vi "实时小时数据单参数上传.vi"(11 "错误输入（无错误）":errorcluster) -> (4 "数据发送起始时间":timestamp format="%<%.3X\n%Y/%m/%d>T", 15 "error out":errorcluster)   [LabVIEW 2016, in "数据传输系统-06.lvlib"]
uses:
  <vilib>/Utility/config.llb/Read Key (String).vi
  <vilib>/Utility/config.llb/Write Key (String).vi
  <vilib>/Utility/config.llb/NI_LVConfig.lvlib
panel:
  out "数据拆分":bool
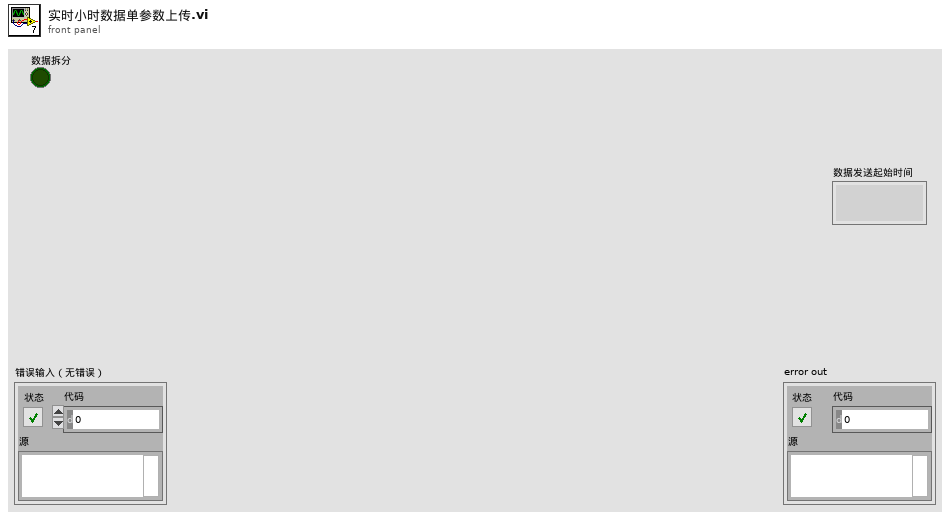
[diagram p1: front panel]
types:
  T1 = cluster{"CODMn":string, "CODCr":string, "DO":string, "铜":string, "PH":string, "氨氮":string, "比电导率":string, "水温":string, "COD":string, "浊度":string, "总氮":string, "总磷":string, "叶绿素a":string, "藻密度":string, "水位":string, "流速":string, "瞬时流量":string, "累积流量":string, "亚硝酸盐":string, "硫化物":string, "ORP":string, "铅":string, "镉":string, "锌":string, "镍":string, "锰":string, "汞":string, "气温":string, "气压":string, "风速":string, "风向":string, "盐度":string, "磷酸盐":string, "硝氮":string, "氟化物":string, "挥发酚":string, "氯化物":string}
  T2 = cluster{"setini":string, "sysini":string, "hechaini":string, "actualwrite":string, "actualread":string, "datasent":string, "反控命令信息队列":string, "反控与仪器交互":string}
  T3 = typedef "NI_LVConfig.lvlib/Config Data RefNum.ctl" = refnum<k1>
  T4 = cluster{"time1":string, "time2":string, "time3":string, "time4":string, "time5":string, "time6":string, "time7":string, "time8":string, "time9":string, "time10":string, "time11":string, "time12":string, "time13":string, "time14":string, "time15":string, "time16":string, "time17":string, "time18":string, "time19":string, "time20":string, "time21":string, "time22":string, "time23":string, "time24":string, "time25":string, "time26":string, "time27":string, "time28":string, "time29":string, "time30":string, "time31":string, "time32":string, "time33":string, "time34":string, "time35":string, "time36":string, "time37":string}
  T5 = cluster{"水样数据索引[0]":string, "水样数据索引[1]":string, "水样数据索引[2]":string, "水样数据索引[3]":string, "水样数据索引[4]":string, "水样数据索引[5]":string, "水样数据索引[6]":string, "水样数据索引[7]":string, "水样数据索引[8]":string, "水样数据索引[9]":string, "水样数据索引[10]":string, "水样数据索引[11]":string, "水样数据索引[12]":string, "水样数据索引[13]":string, "水样数据索引[14]":string, "水样数据索引[15]":string, "水样数据索引[16]":string, "水样数据索引[17]":string, "水样数据索引[18]":string, "水样数据索引[19]":string, "水样数据索引[20]":string, "水样数据索引[21]":string, "水样数据索引[22]":string, "水样数据索引[23]":string, "水样数据索引[24]":string, "水样数据索引[25]":string, "水样数据索引[26]":string, "水样数据索引[27]":string, "水样数据索引[28]":string, "水样数据索引[29]":string, "水样数据索引[30]":string, "水样数据索引[31]":string, "水样数据索引[32]":string, "水样数据索引[33]":string, "水样数据索引[34]":string, "水样数据索引[35]":string, "水样数据索引[36]":string}
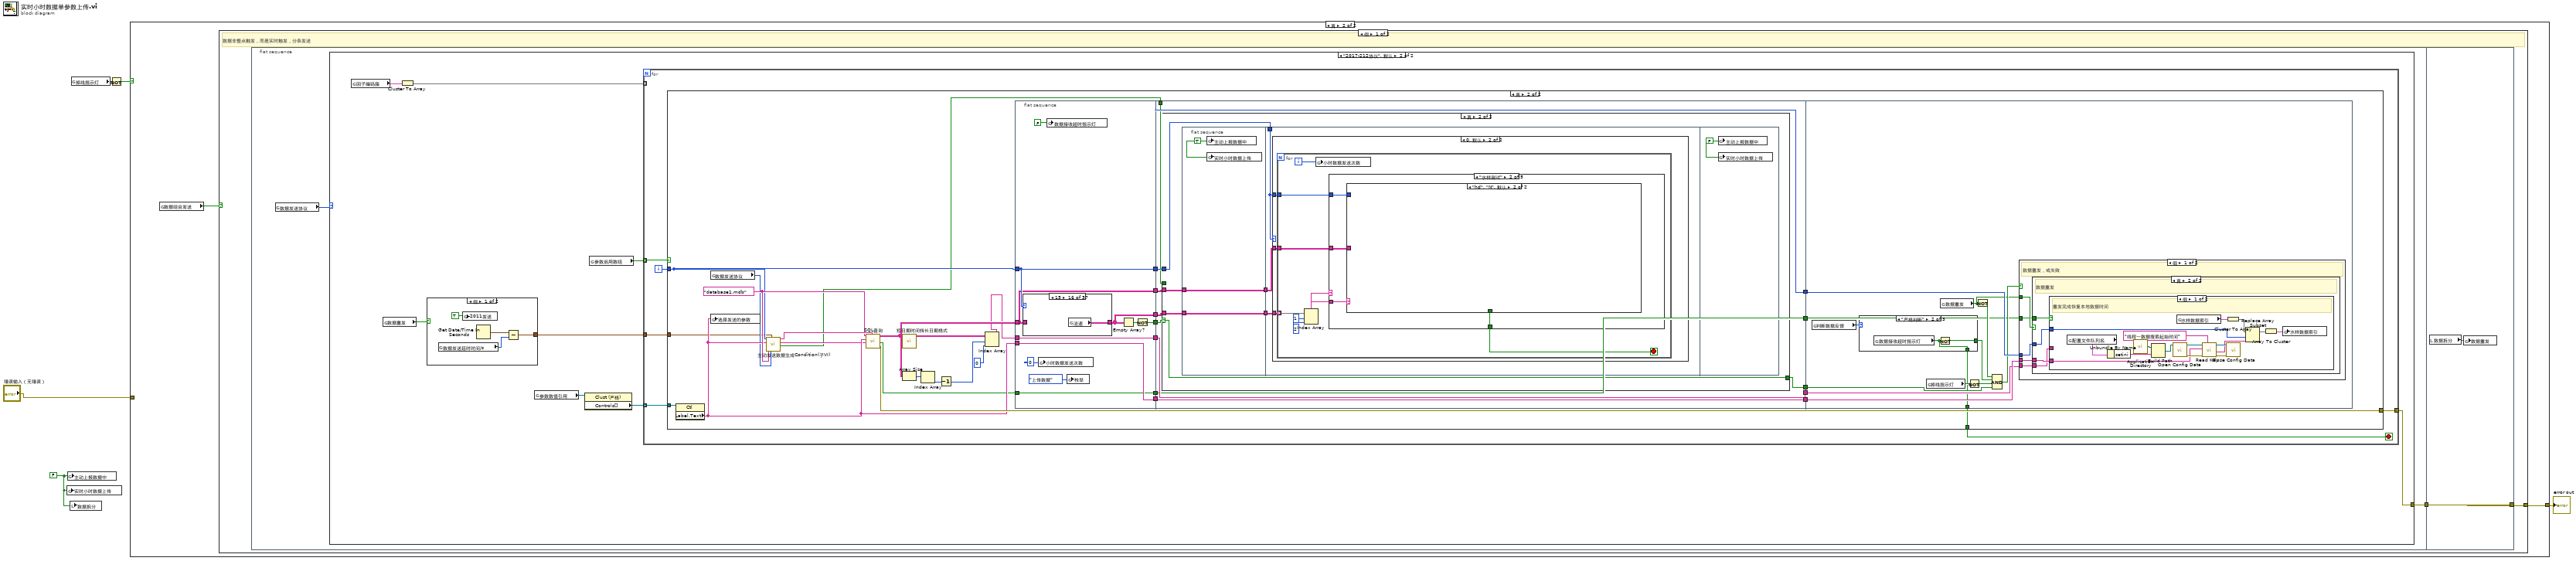
[diagram p0: block diagram]
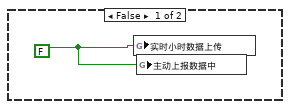
[diagram p2: hidden frame]
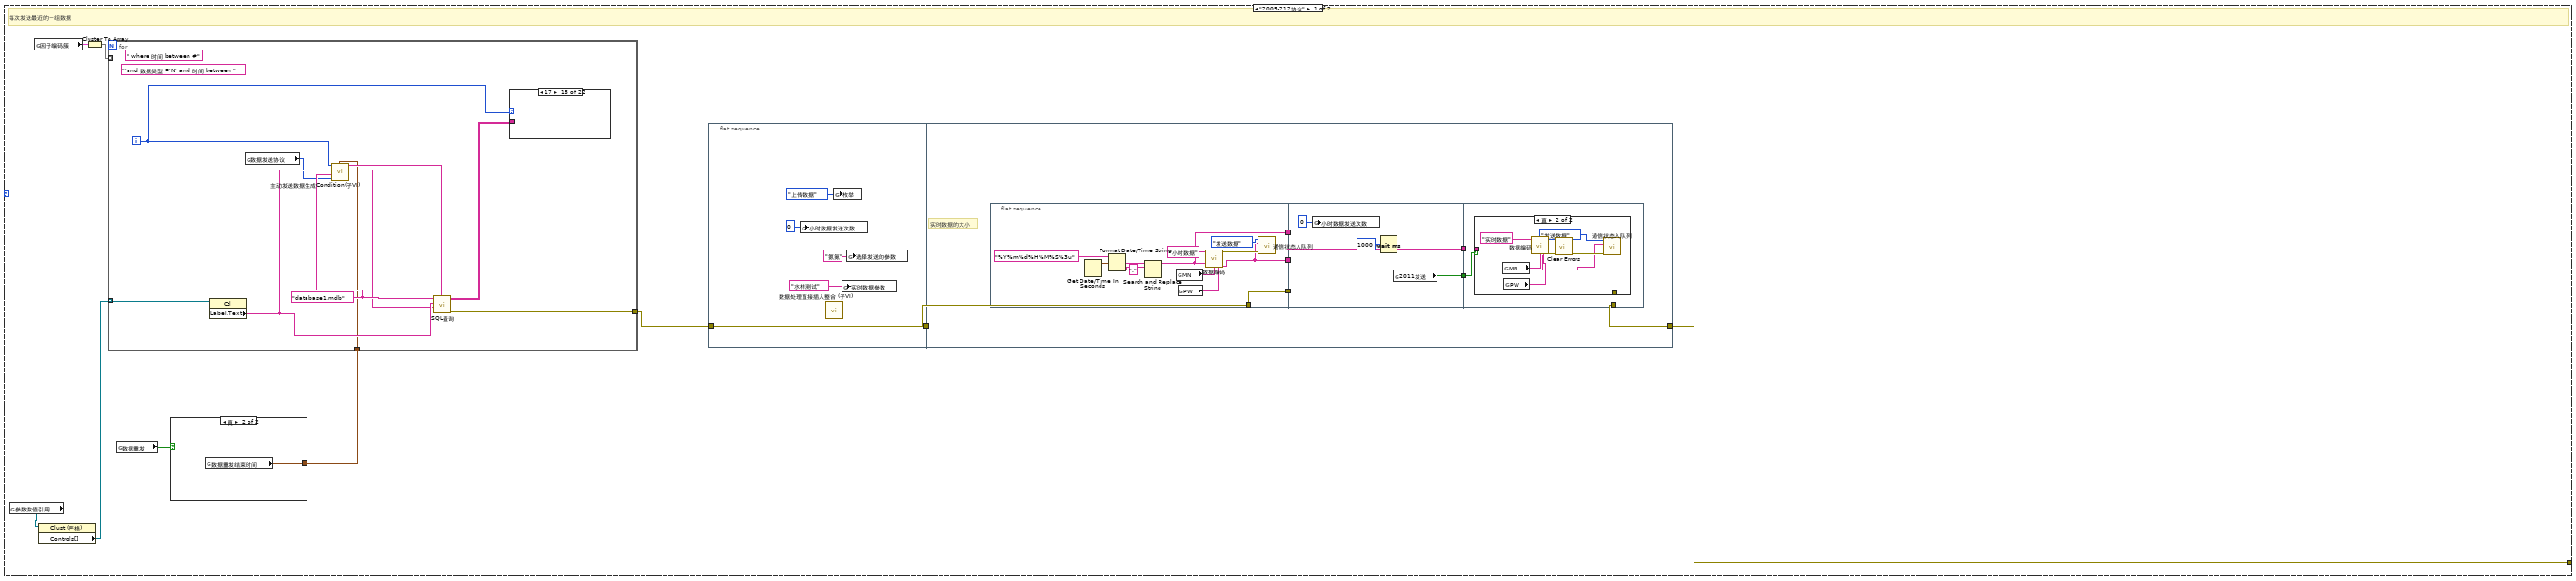
[diagram p3: hidden frame]
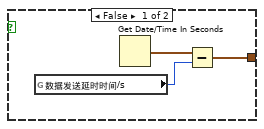
[diagram p4: hidden frame]
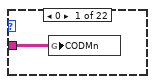
[diagram p6: hidden frame]
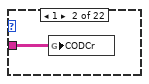
[diagram p7: hidden frame]
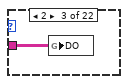
[diagram p8: hidden frame]
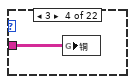
[diagram p9: hidden frame]
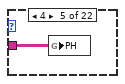
[diagram p10: hidden frame]
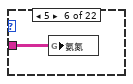
[diagram p11: hidden frame]
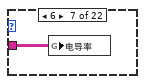
[diagram p12: hidden frame]
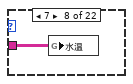
[diagram p13: hidden frame]
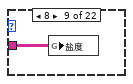
[diagram p14: hidden frame]
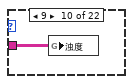
[diagram p15: hidden frame]
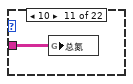
[diagram p16: hidden frame]
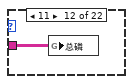
[diagram p17: hidden frame]
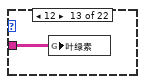
[diagram p18: hidden frame]
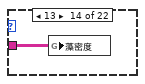
[diagram p19: hidden frame]
diagram:
  w1 = FALSE ("小时数据上传")
  n1 = global write "全局1.vi" "实时小时数据上传"(w1) -> ()
  n2 = global write "全局 数据发送重叠.vi" "主动上报数据中"(w1) -> ()
  n3 = local write "数据拆分"(w1) -> ()
  n4 = global read "全局 数据发送重叠.vi" "掉线指示灯"() -> (w5:bool)
  n5 = Not(x=w5) -> (.not. x?=w4:bool)
  n6 = case shown="真" w4 {
    tunnel: [_ w8] -> w3
    tunnel: "错误输入（无错误）" -> [_ _]
    frame False {
      w6 = FALSE ("小时数据上传")
      n7 = global write "全局1.vi" "实时小时数据上传"(w6) -> ()
      n8 = global write "全局 数据发送重叠.vi" "主动上报数据中"(w6) -> ()
    }
    frame True {
      n9 = global read "断电保存全局.vi" "数据组合发送"() -> (w7:bool)
      n10 = case shown="假" w7 {
        tunnel: [w9 _] -> w8
        frame False {
          # "数据非整点触发，而是实时触发，分条发送"
          n11 = flat-sequence {
            tunnel: [w12] -> w10
            tunnel: [w370] -> w9
            tunnel: w10 -> [w370]
            frame #0 {
              n12 = global read "断电保存全局.vi" "数据发送协议"() -> (w11:enum16{"2005-212协议", "2017-212协议"})
              n13 = case shown="\"2017-212协议\", 默认" w11 {
                tunnel: [w17 w99] -> w12
                frame "2005-212协议" {
                  # "每次发送最近的一组数据"
                  n14 = global read "断电保存全局.vi" "参数数值引用"() -> (w15:refnum<vi>)
                  n15 = global read "断电保存全局.vi" "因子编码簇"() -> (w16:T1)
                  n16 = property class="Clust (严格)"(reference=w15) -> ("Controls[]"=w18:refnum<vi>[])  [unwired: 1 in, 2 out]
                  n17 = Cluster To Array(cluster=w16) -> (array=w21:string[])
                  n18 = global read "断电保存全局.vi" "数据重发"() -> (w14:bool)
                  n19 = case shown="真" w14 {
                    tunnel: [w22 w25] -> w13
                    frame False {
                      n20 = global read "断电保存全局.vi" "数据发送延时时间/s"() -> (w23:i32)
                      n21 = Get Date/Time In Seconds() -> (seconds since 1Jan1904=w24:timestamp)
                      n22 = Subtract(x=w24, y=w23) -> (x-y=w22:timestamp)
                    }
                    frame True {
                      n23 = global read "断电保存全局.vi" "数据重发结束时间"() -> (w25:timestamp)
                    }
                  }
                  n24 = for {
                    tunnel: w21 -> [_] mode=indexing
                    tunnel: [w75] -> w20
                    tunnel: w18 -> [w70] mode=indexing
                    tunnel: w13 -> [w67]
                    i -> [w68]
                    (unwired) " where 时间 between #"
                    w73 = "database1.mdb" ("database")
                    (unwired) "'and 数据类型 ='N' and 时间 between "
                    n25 = property class="Ctl"(reference=w70) -> ("Label.Text"=w74:string)  [unwired: 1 in, 2 out]
                    n26 = global read "断电保存全局.vi" "数据发送协议"() -> (w71:enum16{"2005-212协议", "2017-212协议"})
                    n27 = call "主动发送数据生成Condition(子VI).vi"("结束时间"=w67, "数据发送协议"=w71, "database"=w73, "Label.Text"=w74, "数值"=w68) -> ("columns"=w66:string[], "CONDITION"=w72:string)  [unwired: 3 in, 2 out]
                    n28 = call "SQL查询.vi"("condition"=w72, "columns"=w66, "table输入"=w74, "database"=w73) -> ("error out"=w75:errorcluster, "data"=w69:string[][])  [unwired: 4 in, 2 out]
                    n29 = case shown="17" w68 {
                      tunnel: w69 -> [w76 w77 w78 w79 w80 w81 w82 w83 w84 w85 w86 w87 w88 w89 _ _ _ _ w90 w91 w92 _]
                      frame 0 {
                        n30 = global write "全局 所有参数.vi" "CODMn"(w76) -> ()
                      }
                      frame 1 {
                        n31 = global write "全局 所有参数.vi" "CODCr"(w77) -> ()
                      }
                      frame 2 {
                        n32 = global write "全局 所有参数.vi" "DO"(w78) -> ()
                      }
                      frame 3 {
                        n33 = global write "全局 所有参数.vi" "铜"(w79) -> ()
                      }
                      frame 4 {
                        n34 = global write "全局 所有参数.vi" "PH"(w80) -> ()
                      }
                      frame 5 {
                        n35 = global write "全局 所有参数.vi" "氨氮"(w81) -> ()
                      }
                      frame 6 {
                        n36 = global write "全局 所有参数.vi" "电导率"(w82) -> ()
                      }
                      frame 7 {
                        n37 = global write "全局 所有参数.vi" "水温"(w83) -> ()
                      }
                      frame 8 {
                        n38 = global write "全局 所有参数.vi" "盐度"(w84) -> ()
                      }
                      frame 9 {
                        n39 = global write "全局 所有参数.vi" "浊度"(w85) -> ()
                      }
                      frame 10 {
                        n40 = global write "全局 所有参数.vi" "总氮"(w86) -> ()
                      }
                      frame 11 {
                        n41 = global write "全局 所有参数.vi" "总磷"(w87) -> ()
                      }
                      frame 12 {
                        n42 = global write "全局 所有参数.vi" "叶绿素"(w88) -> ()
                      }
                      frame 13 {
                        n43 = global write "全局 所有参数.vi" "藻密度"(w89) -> ()
                      }
                      frame 14 {
                      }
                      frame 15 {
                      }
                      frame 16 {
                      }
                      frame 17 {
                      }
                      frame 18 {
                        n44 = global write "全局 所有参数.vi" "亚硝酸盐"(w90) -> ()
                      }
                      frame 19 {
                        n45 = global write "全局 所有参数.vi" "硫化物"(w91) -> ()
                      }
                      frame 20 {
                        n46 = global write "全局 所有参数.vi" "ORP"(w92) -> ()
                      }
                      frame 21, Default {
                      }
                    }
                  }
                  n47 = flat-sequence {
                    tunnel: w20 -> [w26]
                    tunnel: [w26] -> w19
                    tunnel: w19 -> [w35]
                    tunnel: [w34] -> w17
                    frame #0 {
                      n48 = global write "全局 小时数据发送次数.vi" "小时数据发送次数"(0 ("小时数据发送次数")) -> ()
                      n49 = call "数据处理直接插入整合 (子VI).vi"() -> ()  [unwired: 12 in]
                      n50 = global write "全局1.vi" "枚举"(enum16{"返回请求应答", "上传数据", "返回执行结果"}."上传数据" ("枚举")) -> ()
                      n51 = global write "全局 实时数据参数.vi" "实时数据参数"("水样测试" ("实时数据参数")) -> ()
                      n52 = global write "全局 水样时间.vi" "选择发送的参数"("氨氮" ("选择发送的参数")) -> ()
                    }
                    frame #1 {
                      # "实时数据的大小"
                      n53 = flat-sequence {
                        tunnel: [w38] -> w37
                        tunnel: [w41] -> w36
                        tunnel: w35 -> [w41]
                        tunnel: [w40] -> w33
                        tunnel: w37 -> [_]
                        tunnel: w36 -> [_]
                        tunnel: w33 -> [w51]
                        tunnel: [w51] -> w32
                        tunnel: [w50] -> w31
                        tunnel: [w56] -> w34
                        tunnel: w32 -> [w55]
                        tunnel: w31 -> [w54]
                        frame #0 {
                          n54 = Get Date/Time In Seconds() -> (seconds since 1Jan1904=w47:timestamp)
                          n55 = Format Date/Time String(time format string (%c)="%Y%m%d%H%M%S%3u" ("时间格式字符串(%c)"), seconds (now)=w47) -> (date/time string=w48:string)  [unwired: 1 in]
                          n56 = Search and Replace String(input string=w48, search string="." ("搜索字符串")) -> (result string=w40:string)  [unwired: 6 in, 3 out]
                          n57 = global read "断电保存全局.vi" "MN"() -> (w44:string)
                          n58 = global read "断电保存全局.vi" "PW"() -> (w43:string)
                          n59 = call "数据编码.vi"("table输入"="小时数据" ("新元素/子数组"), "QN"=w40, "MN"=w44, "PW"=w43) -> ("错误常量"=w42:errorcluster, "通讯包字符串"=w38:string)  [unwired: 10 in]
                          n60 = call "通信状态入队列.vi"("错误输入（无错误）"=w42, "发送报文"=w38, "枚举"=enum16{"打开连接", "发送数据", "读取数据", "数据处理", "关闭连接"}."发送数据") -> ()  [unwired: 8 in, 1 out]
                        }
                        frame #1 {
                          n61 = global write "全局 小时数据发送次数.vi" "小时数据发送次数"(0 ("小时数据发送次数")) -> ()
                          n62 = Wait (ms)(milliseconds to wait=u32 1000 ("等待时间（毫秒）")) -> ()  [unwired: 1 out]
                          n63 = global read "断电保存全局.vi" "2011发送"() -> (w50:bool)
                        }
                        frame #2 {
                          n64 = case shown="真" w54 {
                            tunnel: [_ w61] -> w56
                            tunnel: w55 -> [_ w60]
                            frame False {
                            }
                            frame True {
                              n65 = global read "断电保存全局.vi" "MN"() -> (w63:string)
                              n66 = global read "断电保存全局.vi" "PW"() -> (w64:string)
                              n67 = call "数据编码.vi"("table输入"="实时数据" ("新元素/子数组"), "QN"=w60, "MN"=w63, "PW"=w64) -> ("错误常量"=w62:errorcluster, "通讯包字符串"=w57:string)  [unwired: 10 in]
                              n68 = call <vilib>:"Clear Errors.vi"("error in (no error)"=w62) -> ("error out"=w59:errorcluster)  [unwired: 5 in, 1 out]
                              n69 = call "通信状态入队列.vi"("错误输入（无错误）"=w59, "发送报文"=w57, "枚举"=enum16{"打开连接", "发送数据", "读取数据", "数据处理", "关闭连接"}."发送数据") -> ("错误输出"=w61:errorcluster)  [unwired: 8 in]
                            }
                          }
                        }
                      }
                    }
                  }
                }
                frame "2017-212协议", Default {
                  n70 = global read "断电保存全局.vi" "因子编码簇"() -> (w97:T1)
                  n71 = global read "断电保存全局.vi" "数据重发"() -> (w94:bool)
                  n72 = Cluster To Array(cluster=w97) -> (array=w100:string[])
                  n73 = case shown="假" w94 {
                    tunnel: [w102 w105] -> w93
                    frame False {
                      n74 = global read "断电保存全局.vi" "数据发送延时时间/s"() -> (w103:i32)
                      n75 = global write "断电保存全局.vi" "2011发送"(TRUE ("2011发送")) -> ()
                      n76 = Get Date/Time In Seconds() -> (seconds since 1Jan1904=w104:timestamp)
                      n77 = Subtract(x=w104, y=w103) -> (x-y=w102:timestamp)
                    }
                    frame True {
                      n78 = global read "断电保存全局.vi" "数据重发结束时间"() -> (w105:timestamp)
                    }
                  }
                  n79 = global read "断电保存全局.vi" "参数数值引用"() -> (w96:refnum<vi>)
                  n80 = property class="Clust (严格)"(reference=w96) -> ("Controls[]"=w98:refnum<vi>[])  [unwired: 1 in, 2 out]
                  n81 = global read "断电保存全局.vi" "参数启用数组"() -> (w95:bool[])
                  n82 = for {
                    tunnel: w100 -> [_] mode=indexing
                    tunnel: [w111] -> w99
                    tunnel: w98 -> [w109] mode=indexing
                    tunnel: w95 -> [w108] mode=indexing
                    tunnel: w93 -> [w107]
                    i -> [w110]
                    stop <- w106 stop-if-true
                    n83 = case shown="真" w108 {
                      tunnel: [_ w132] -> w111
                      tunnel: w110 -> [_ w123]
                      tunnel: w109 -> [_ w122]
                      tunnel: w107 -> [_ w119]
                      tunnel: [_ w117] -> w106
                      frame False {
                      }
                      frame True {
                        w131 = "database1.mdb" ("database")
                        n84 = property class="Ctl"(reference=w122) -> ("Label.Text"=w130:string)  [unwired: 1 in, 2 out]
                        n85 = global read "断电保存全局.vi" "数据发送协议"() -> (w129:enum16{"2005-212协议", "2017-212协议"})
                        n86 = global write "全局 水样时间.vi" "选择发送的参数"(w130) -> ()
                        n87 = call "主动发送数据生成Condition(子VI).vi"("结束时间"=w119, "数据发送协议"=w129, "database"=w131, "Label.Text"=w130, "数值"=w123) -> ("database溢出"=w112:bool, "columns"=w121:string[], "CONDITION"=w134:string)  [unwired: 3 in, 1 out]
                        n88 = call "SQL查询.vi"("condition"=w134, "columns"=w121, "table输入"=w130, "database"=w131) -> ("error out"=w132:errorcluster, "拆分数据"=w115:bool, "data"=w126:string[][])  [unwired: 4 in, 1 out]
                        n89 = call "短日期时间转长日期格式.vi"("data"=w126) -> ("输出数组"=w133:string[][])  [unwired: 10 in]
                        n90 = Array Size(array=w126) -> (size(s)=w128:i32[])
                        n91 = Index Array(array=w128) -> (element=w127:i32)  [unwired: 1 in]
                        n92 = Decrement(x=w127) -> (x-1=w125:i32)
                        n93 = Index Array(array=w133, index (row)=w125, index (col)=0 ("禁用的索引 (列)")) -> (element=w113:string)
                        n94 = flat-sequence {
                          tunnel: [w146] -> w142
                          tunnel: [w145] -> w141
                          tunnel: w126 -> [w144]
                          tunnel: w123 -> [w149]
                          tunnel: w130 -> [w151]
                          tunnel: [w151] -> w140
                          tunnel: w113 -> [w150]
                          tunnel: [w150] -> w139
                          tunnel: [w149] -> w138
                          tunnel: [w144] -> w118
                          tunnel: [w143] -> w116
                          tunnel: w115 -> [w143]
                          tunnel: w142 -> [w195]
                          tunnel: w141 -> [w199]
                          tunnel: [w198] -> w137
                          tunnel: w140 -> [w198]
                          tunnel: [w197] -> w136
                          tunnel: w139 -> [w197]
                          tunnel: [w196] -> w135
                          tunnel: w138 -> [w196]
                          tunnel: [w192] -> w120
                          tunnel: w118 -> [w194]
                          tunnel: w116 -> [w193]
                          tunnel: [w193] -> w114
                          tunnel: w112 -> [w191]
                          tunnel: w137 -> [w310]
                          tunnel: w136 -> [w309]
                          tunnel: w135 -> [w308]
                          tunnel: w120 -> [w307]
                          tunnel: [w299] -> w117
                          tunnel: w114 -> [w298]
                          frame #0 {
                            n95 = case shown="15" w149 {
                              tunnel: w144 -> [w154 w155 w156 w157 w158 w159 w160 w161 w162 w163 w164 w165 w166 w167 _ _ _ _ w172 w173 w174 w175 w176 w177 w178 w179 w180 _ _ _ _ w185 w186 w187 w188 w189 w190]
                              tunnel: [w154 w155 w156 w157 w158 w159 w160 w161 w162 w163 w164 w165 w166 w167 w168 w169 w170 w171 w172 w173 w174 w175 w176 w177 w178 w179 w180 w181 w182 w183 w184 w185 w186 w187 w188 w189 w190] -> w145
                              frame 0, Default {
                                n96 = global write "全局 所有参数.vi" "CODMn"(w154) -> ()
                              }
                              frame 1 {
                                n97 = global write "全局 所有参数.vi" "CODCr"(w155) -> ()
                              }
                              frame 2 {
                                n98 = global write "全局 所有参数.vi" "DO"(w156) -> ()
                              }
                              frame 3 {
                                n99 = global write "全局 所有参数.vi" "铜"(w157) -> ()
                              }
                              frame 4 {
                                n100 = global write "全局 所有参数.vi" "PH"(w158) -> ()
                              }
                              frame 5 {
                                n101 = global write "全局 所有参数.vi" "氨氮"(w159) -> ()
                              }
                              frame 6 {
                                n102 = global write "全局 所有参数.vi" "电导率"(w160) -> ()
                              }
                              frame 7 {
                                n103 = global write "全局 所有参数.vi" "水温"(w161) -> ()
                              }
                              frame 8 {
                                n104 = global write "全局 所有参数.vi" "盐度"(w162) -> ()
                              }
                              frame 9 {
                                n105 = global write "全局 所有参数.vi" "浊度"(w163) -> ()
                              }
                              frame 10 {
                                n106 = global write "全局 所有参数.vi" "总氮"(w164) -> ()
                              }
                              frame 11 {
                                n107 = global write "全局 所有参数.vi" "总磷"(w165) -> ()
                              }
                              frame 12 {
                                n108 = global write "全局 所有参数.vi" "叶绿素"(w166) -> ()
                              }
                              frame 13 {
                                n109 = global write "全局 所有参数.vi" "藻密度"(w167) -> ()
                              }
                              frame 14 {
                                n110 = global read "全局 所有参数.vi" "水位"() -> (w168:string[][])
                              }
                              frame 15 {
                                n111 = global read "全局 所有参数.vi" "流速"() -> (w169:string[][])
                              }
                              frame 16 {
                                n112 = global read "全局 所有参数.vi" "瞬时流量"() -> (w170:string[][])
                              }
                              frame 17 {
                                n113 = global read "全局 所有参数.vi" "累积流量"() -> (w171:string[][])
                              }
                              frame 18 {
                                n114 = global write "全局 所有参数.vi" "亚硝酸盐"(w172) -> ()
                              }
                              frame 19 {
                                n115 = global write "全局 所有参数.vi" "硫化物"(w173) -> ()
                              }
                              frame 20 {
                                n116 = global write "全局 所有参数.vi" "ORP"(w174) -> ()
                              }
                              frame 21 {
                                n117 = global write "全局 所有参数.vi" "铅"(w175) -> ()
                              }
                              frame 22 {
                                n118 = global write "全局 所有参数.vi" "镉"(w176) -> ()
                              }
                              frame 23 {
                                n119 = global write "全局 所有参数.vi" "锌"(w177) -> ()
                              }
                              frame 24 {
                                n120 = global write "全局 所有参数.vi" "镍"(w178) -> ()
                              }
                              frame 25 {
                                n121 = global write "全局 所有参数.vi" "锰"(w179) -> ()
                              }
                              frame 26 {
                                n122 = global write "全局 所有参数.vi" "汞"(w180) -> ()
                              }
                              frame 27 {
                                n123 = global read "全局 所有参数.vi" "气温"() -> (w181:string[][])
                              }
                              frame 28 {
                                n124 = global read "全局 所有参数.vi" "气压"() -> (w182:string[][])
                              }
                              frame 29 {
                                n125 = global read "全局 所有参数.vi" "风速"() -> (w183:string[][])
                              }
                              frame 30 {
                                n126 = global read "全局 所有参数.vi" "风向"() -> (w184:string[][])
                              }
                              frame 31 {
                                n127 = global write "全局 所有参数.vi" "盐度 2"(w185) -> ()
                              }
                              frame 32 {
                                n128 = global write "全局 所有参数.vi" "磷酸盐"(w186) -> ()
                              }
                              frame 33 {
                                n129 = global write "全局 所有参数.vi" "硝氮"(w187) -> ()
                              }
                              frame 34 {
                                n130 = global write "全局 所有参数.vi" "氟化物"(w188) -> ()
                              }
                              frame 35 {
                                n131 = global write "全局 所有参数.vi" "挥发酚"(w189) -> ()
                              }
                              frame 36 {
                                n132 = global write "全局 所有参数.vi" "氯化物"(w190) -> ()
                              }
                            }
                            n133 = global write "全局 小时数据发送次数.vi" "小时数据发送次数"(0 ("小时数据发送次数")) -> ()
                            n134 = global write "全局 数据发送重叠.vi" "数据接收超时指示灯"(FALSE ("数据接收超时指示灯")) -> ()
                            n135 = global write "全局1.vi" "枚举"(enum16{"返回请求应答", "上传数据", "返回执行结果"}."上传数据" ("枚举")) -> ()
                            n136 = Empty Array?(array=w145) -> (empty?=w147:bool)
                            n137 = Not(x=w147) -> (.not. x?=w146:bool)
                          }
                          frame #1 {
                            n138 = case shown="真" w195 {
                              selector: w195 -> [_ w201]
                              tunnel: w199 -> [_ w206]
                              tunnel: w196 -> [_ w205]
                              tunnel: w194 -> [_ w203]
                              tunnel: [w200 w201] -> w192
                              tunnel: w191 -> [w200 _]
                              frame False {
                              }
                              frame True {
                                n139 = flat-sequence {
                                tunnel: w206 -> [w209]
                                tunnel: [w209] -> w204
                                tunnel: w203 -> [w207]
                                tunnel: [w207] -> w202
                                tunnel: w205 -> [w211]
                                tunnel: w204 -> [w212]
                                tunnel: w202 -> [w210]
                                frame #0 {
                                w208 = TRUE ("小时数据上传")
                                n140 = global write "全局 数据发送重叠.vi" "主动上报数据中"(w208) -> ()
                                n141 = global write "全局1.vi" "实时小时数据上传"(w208) -> ()
                                }
                                frame #1 {
                                n142 = case shown="0, 默认" w211 {
                                selector: w211 -> [w213 _]
                                tunnel: w211 -> [_ w244]
                                tunnel: w212 -> [w216 w243]
                                tunnel: w210 -> [w215 w242]
                                frame 14..17, 27..30 {
                                n143 = for {
                                tunnel: [w240] -> w217
                                tunnel: w213 -> [w239]
                                tunnel: w216 -> [_] mode=indexing
                                i -> [w241]
                                stop <- w238 stop-if-true
                                n144 = call "小时数据发送 (子VI).vi"("数值"=w239) -> ("error out"=w240:errorcluster, "超时退出"=w238:bool)  [unwired: 9 in]
                                n145 = global write "全局 小时数据发送次数.vi" "小时数据发送次数"(w241) -> ()
                                }
                                n146 = global read "断电保存全局.vi" "2011发送"() -> (w214:bool)
                                n147 = case shown="真" w214 {
                                tunnel: w217 -> [_ w222]
                                tunnel: w213 -> [_ w221]
                                tunnel: w215 -> [_ w220]
                                tunnel: w213 -> [_ w218]
                                frame False {
                                }
                                frame True {
                                n148 = flat-sequence {
                                tunnel: w222 -> [w226]
                                tunnel: [w226] -> w223
                                tunnel: w221 -> [w225]
                                tunnel: w220 -> [w224]
                                tunnel: [w224] -> w219
                                frame #0 {
                                n149 = case shown="27" w225 {
                                tunnel: w224 -> [_ w227 w228 w229 w230 w231 w232 w233 w234]
                                frame 0, Default {
                                }
                                frame 14 {
                                n150 = global write "全局 所有参数.vi" "水位"(w227) -> ()
                                }
                                frame 15 {
                                n151 = global write "全局 所有参数.vi" "流速"(w228) -> ()
                                }
                                frame 16 {
                                n152 = global write "全局 所有参数.vi" "瞬时流量"(w229) -> ()
                                }
                                frame 17 {
                                n153 = global write "全局 所有参数.vi" "累积流量"(w230) -> ()
                                }
                                frame 27 {
                                n154 = global write "全局 所有参数.vi" "气温"(w231) -> ()
                                }
                                frame 28 {
                                n155 = global write "全局 所有参数.vi" "气压"(w232) -> ()
                                }
                                frame 29 {
                                n156 = global write "全局 所有参数.vi" "风速"(w233) -> ()
                                }
                                frame 30 {
                                n157 = global write "全局 所有参数.vi" "风向"(w234) -> ()
                                }
                                }
                                }
                                }
                                n158 = for {
                                tunnel: w223 -> [_]
                                tunnel: w219 -> [_] mode=indexing
                                tunnel: w218 -> [w236]
                                i -> [w237]
                                stop <- w235 stop-if-true
                                n159 = global write "全局 小时数据发送次数.vi" "小时数据发送次数"(w237) -> ()
                                n160 = call "实时数据发送 (子VI).vi"("数值"=w236) -> ("超时退出"=w235:bool)  [unwired: 10 in]
                                }
                                }
                                }
                                }
                                frame 0, Default {
                                n161 = for {
                                tunnel: w244 -> [w247]
                                tunnel: w243 -> [w253] mode=indexing
                                tunnel: w242 -> [w249]
                                i -> [w248]
                                stop <- w245 stop-if-true
                                n162 = Index Array(array=w253, index #1=1 ("索引"), index #2=2 ("索引")) -> (element #1=w246:string, element #2=w250:string)
                                n163 = global write "全局 小时数据发送次数.vi" "小时数据发送次数"(w248) -> ()
                                n164 = case shown="\"水样测试\"" w246 {
                                tunnel: w247 -> [_ w257 _ _ _]
                                tunnel: w250 -> [_ w256 w289 w292 w295]
                                tunnel: w249 -> [_ w255 _ _ _]
                                tunnel: [_ w254 w288 w291 w294] -> w245
                                frame "假", Default {
                                }
                                frame "水样测试" {
                                n165 = case shown="\"hd\", \"N\", 默认" w256 {
                                tunnel: w257 -> [w261 w282]
                                tunnel: w255 -> [w260 w281]
                                tunnel: [w258 w279] -> w254
                                frame "M" {
                                n166 = global read "断电保存全局.vi" "2011发送"() -> (w259:bool)
                                n167 = case shown="真" w259 {
                                tunnel: w261 -> [_ w264]
                                tunnel: w260 -> [_ w263]
                                tunnel: [_ w262] -> w258
                                frame False {
                                }
                                frame True {
                                n168 = flat-sequence {
                                tunnel: w264 -> [w266]
                                tunnel: w263 -> [w267]
                                tunnel: [w266] -> w265
                                tunnel: w265 -> [w277]
                                tunnel: [w276] -> w262
                                frame #0 {
                                n169 = case shown="14" w266 {
                                tunnel: w267 -> [_ w268 w269 w270 w271 w272 w273 w274 w275]
                                frame 0, Default {
                                }
                                frame 14 {
                                n170 = global write "全局 所有参数.vi" "水位"(w268) -> ()
                                }
                                frame 15 {
                                n171 = global write "全局 所有参数.vi" "流速"(w269) -> ()
                                }
                                frame 16 {
                                n172 = global write "全局 所有参数.vi" "瞬时流量"(w270) -> ()
                                }
                                frame 17 {
                                n173 = global write "全局 所有参数.vi" "累积流量"(w271) -> ()
                                }
                                frame 27 {
                                n174 = global write "全局 所有参数.vi" "气温"(w272) -> ()
                                }
                                frame 28 {
                                n175 = global write "全局 所有参数.vi" "气压"(w273) -> ()
                                }
                                frame 29 {
                                n176 = global write "全局 所有参数.vi" "风速"(w274) -> ()
                                }
                                frame 30 {
                                n177 = global write "全局 所有参数.vi" "风向"(w275) -> ()
                                }
                                }
                                }
                                frame #1 {
                                n178 = call "实时数据发送 (子VI).vi"("数值"=w277) -> ("超时退出"=w276:bool)  [unwired: 10 in]
                                }
                                }
                                }
                                }
                                }
                                frame "hd", "N", Default {
                                n179 = call "小时数据发送 (子VI).vi"("数值"=w282) -> ("error out"=w280:errorcluster, "超时退出"=w278:bool)  [unwired: 9 in]
                                n180 = global read "断电保存全局.vi" "2011发送"() -> (w283:bool)
                                n181 = case shown="真" w283 {
                                tunnel: w282 -> [_ w287]
                                tunnel: w281 -> [_ _]
                                tunnel: w280 -> [_ _]
                                tunnel: [_ w284] -> w279
                                tunnel: w278 -> [_ w286]
                                frame False {
                                }
                                frame True {
                                n182 = call "实时数据发送 (子VI).vi"("数值"=w287) -> ("超时退出"=w285:bool)  [unwired: 10 in]
                                n183 = Or(x=w286, y=w285) -> (x .or. y?=w284:bool)
                                }
                                }
                                }
                                }
                                }
                                frame "空白测试", "零点核查" {
                                n184 = case shown="\"N\", 默认" w289 {
                                tunnel: [_ w290] -> w288
                                frame "M" {
                                }
                                frame "N", Default {
                                n185 = call "零点核查数据发送 (子VI).vi"() -> ("超时退出"=w290:bool)  [unwired: 11 in]
                                }
                                }
                                }
                                frame "跨度核查" {
                                n186 = case shown="\"N\", 默认" w292 {
                                tunnel: [_ w293] -> w291
                                frame "M" {
                                }
                                frame "N", Default {
                                n187 = call "跨度核查数据发送 (子VI).vi"() -> ("超时退出"=w293:bool)  [unwired: 11 in]
                                }
                                }
                                }
                                frame "标样核查" {
                                n188 = case shown="\"N\", 默认" w295 {
                                tunnel: [_ w296] -> w294
                                frame "M" {
                                }
                                frame "N", Default {
                                n189 = call "标样核查数据发送(子VI).vi"() -> ("超时退出"=w296:bool)  [unwired: 11 in]
                                }
                                }
                                }
                                }
                                }
                                }
                                }
                                }
                                frame #2 {
                                w297 = FALSE ("小时数据上传")
                                n190 = global write "全局 数据发送重叠.vi" "主动上报数据中"(w297) -> ()
                                n191 = global write "全局1.vi" "实时小时数据上传"(w297) -> ()
                                }
                                }
                              }
                            }
                          }
                          frame #2 {
                            n192 = global read "断电保存全局.vi" "判断数据反馈"() -> (w304:enum16{"非严格判断", "严格判断", "不判断"})
                            n193 = case shown="\"严格判断\"" w304 {
                              tunnel: [TRUE w314 TRUE] -> w303
                              tunnel: [FALSE ("数据接收超时指示灯") w313 FALSE ("数据接收超时指示灯")] -> w299
                              frame "非严格判断", Default {
                              }
                              frame "严格判断" {
                                n194 = global read "全局 数据发送重叠.vi" "数据接收超时指示灯"() -> (w313:bool)
                                n195 = Not(x=w313) -> (.not. x?=w314:bool)
                              }
                              frame "不判断" {
                              }
                            }
                            n196 = global read "全局 数据发送重叠.vi" "掉线指示灯"() -> (w306:bool)
                            n197 = global read "断电保存全局.vi" "数据重发"() -> (w300:bool)
                            n198 = Not(x=w306) -> (.not. x?=w305:bool)
                            n199 = Not(x=w300) -> (.not. x?=w301:bool)
                            n200 = Compound Arithmetic op=AND ("复合运算")(w301, w303, w305, w307) -> (w302:bool)
                            n201 = case shown="假" w302 {
                              tunnel: w309 -> [w317 w360]
                              tunnel: w308 -> [w319 w354]
                              tunnel: w310 -> [w321 w361]
                              tunnel: w300 -> [w320 _]
                              tunnel: w298 -> [w318 _]
                              frame False {
                                # "数据重发，或失败"
                                n202 = case shown="真" w320 {
                                tunnel: w321 -> [_ w325]
                                tunnel: w319 -> [_ w324]
                                tunnel: w318 -> [_ w323]
                                tunnel: w317 -> [_ w322]
                                frame False {
                                # "数据发送失败"
                                }
                                frame True {
                                # "数据重发"
                                n203 = case shown="假" w323 {
                                tunnel: w325 -> [w329 _]
                                tunnel: w324 -> [w327 w343]
                                tunnel: w322 -> [_ w344]
                                frame False {
                                # "重发完成恢复本地数据时间"
                                n204 = global read "全局1.vi" "配置文件队列名"() -> (w326:T2)
                                n205 = Unbundle By Name(w326) -> ("setini"=w336:string)
                                n206 = call <vilib>:"Application Directory.vi"() -> ("Application Directory"=w330:path)
                                n207 = Build Path(base path=w330, name or relative path=w336) -> (appended path=w331:path)
                                n208 = call <vilib>:"Open Config Data.vi"("configuration file path"=w331) -> ("error out"=w337:errorcluster, "refnum"=w332:T3)  [unwired: 8 in, 1 out]
                                n209 = global read "全局 水样时间.vi" "水样数据索引"() -> (w338:T4)
                                n210 = call-poly <vilib>:"Read Key.vi"("section"="线程一数据搜索起始时间", "error in (no error)"=w337, "key"=w329, "refnum"=w332) -> ("error out"=w335:errorcluster, "value"=w328:string, "refnum out"=w334:T3)  [unwired: 4 in, 1 out]
                                n211 = Cluster To Array(cluster=w338) -> (array=w339:string[])
                                n212 = call <vilib>:"Close Config Data.vi"("error in (no error)"=w335, "refnum"=w334) -> ()  [unwired: 8 in, 2 out]
                                n213 = Replace Array Subset(array=w339, new element=w328, index=w327) -> (w340:string[])
                                n214 = Array To Cluster(array=w340) -> (cluster=w341:T5)
                                n215 = global write "全局 水样时间.vi" "水样数据索引"(w341) -> ()
                                }
                                frame True {
                                # "数据拆分，继续重发"
                                n216 = call "日期时间字符串转换分钟数加一.vi"("data[0]"=w344) -> ("日期/时间字符串"=w342:string)  [unwired: 10 in]
                                n217 = global read "全局 水样时间.vi" "水样数据索引"() -> (w345:T4)
                                n218 = Cluster To Array(cluster=w345) -> (array=w346:string[])
                                n219 = Replace Array Subset(array=w346, new element=w342, index=w343) -> (w347:string[])
                                n220 = Array To Cluster(array=w347) -> (cluster=w348:T5)
                                n221 = global write "全局 水样时间.vi" "水样数据索引"(w348) -> ()
                                "数据拆分" <- TRUE
                                }
                                }
                                }
                                }
                              }
                              frame True {
                                # "保存本地"
                                n222 = global read "全局1.vi" "配置文件队列名"() -> (w350:T2)
                                n223 = call "日期时间字符串转换分钟数加一.vi"("枚举"=enum16{"分钟数加一", "秒数加一", "小时数加一"}."秒数加一", "data[0]"=w360) -> ("日期/时间字符串"=w353:string)  [unwired: 9 in]
                                n224 = Unbundle By Name(w350) -> ("setini"=w351:string)
                                n225 = global read "全局 水样时间.vi" "水样数据索引"() -> (w355:T4)
                                n226 = call <vilib>:"Application Directory.vi"() -> ("Application Directory"=w362:path)
                                n227 = Build Path(base path=w362, name or relative path=w351) -> (appended path=w363:path)
                                n228 = Cluster To Array(cluster=w355) -> (array=w356:string[])
                                n229 = call <vilib>:"Open Config Data.vi"("configuration file path"=w363) -> ("error out"=w365:errorcluster, "refnum"=w364:T3)  [unwired: 8 in, 1 out]
                                n230 = call "时间日期字符串至时间标识转换.vi"("时间日期字符串"=w353) -> ("时间标识"=→"数据发送起始时间":timestamp)  [unwired: 10 in]
                                n231 = call-poly <vilib>:"Write Key.vi"("section"="线程一数据搜索起始时间", "error in (no error)"=w365, "value"=w353, "key"=w361, "refnum"=w364) -> ("error out"=w367:errorcluster, "refnum out"=w366:T3)  [unwired: 4 in, 1 out]
                                n232 = Replace Array Subset(array=w356, new element=w353, index=w354) -> (w357:string[])
                                n233 = Array To Cluster(array=w357) -> (cluster=w358:T5)
                                n234 = call <vilib>:"Close Config Data.vi"("error in (no error)"=w367, "refnum"=w366) -> ()  [unwired: 8 in, 2 out]
                                n235 = global write "全局 水样时间.vi" "水样数据索引"(w358) -> ()
                              }
                            }
                          }
                        }
                      }
                    }
                  }
                }
              }
            }
            frame #1 {
              n236 = local read "数据拆分"() -> (w369:bool)
              n237 = global write "断电保存全局.vi" "数据重发"(w369) -> ()
            }
          }
        }
        frame True {
          # "数据整点触发，整条发送"
          n238 = flat-sequence {
            frame #0 {
              n239 = global read "断电保存全局.vi" "数据发送通道"() -> (w371:enum16{"TCP", "VISA"})
              n240 = global read "断电保存全局.vi" "MN"() -> (w373:string)
              n241 = global read "断电保存全局.vi" "PW"() -> (w372:string)
              n242 = call "数据全参数一起发送整点触发.vi"("数据发送通道"=w371, "PW"=w372, "MN"=w373) -> ()  [unwired: 8 in]
            }
            frame #1 {
              w374 = FALSE ("主动上报数据中")
              n243 = global write "全局 数据发送重叠.vi" "主动上报数据中"(w374) -> ()
              n244 = global write "全局1.vi" "实时小时数据上传"(w374) -> ()
            }
          }
        }
      }
    }
  }
  "error out" <- w3
